vi "gRPC Client Test.vi"() -> ()   [LabVIEW 2021]
uses:
  CIFCore/Common/Typedef/gRPC Reported Plugin Status.ctl
  CIFCore/Common/Typedef/Plugin State.ctl
  CIFCore/Common/Typedef/Timing Statistics.ctl
  CIFCore/Common/Typedef/Timing Stats Base.ctl
  CIFCore/Common/Typedef/FIFO Statistics.ctl
  CIFCore/Common/Typedef/Simple Error.ctl
  CIFCore/Common/Typedef/Monitor Doubles.ctl
  CIFCore/Common/Typedef/Monitor U64.ctl
  CIFCore/Common/Typedef/Monitor I64.ctl
  CIFCore/Common/Typedef/Version.ctl
  CIFCore/Grpc/CIFCorePlugin_client/RPC Messages/cif_plugincore_PluginOverrides.ctl
  CIFCore/Grpc/CIFCorePlugin_client/RPC Messages/cif_plugincore_TimingOverrides.ctl
  CIFCore/Grpc/CIFCorePluginWrapper/CIFCorePluginWrapper.lvlib
  CIFCore/Common/CIFCoreCommon.lvlib
  CIFCore/Grpc/CIFCorePlugin_client/CIFCorePlugin_client.lvlib
panel:
  in  "JSON Configuration 2":string
  in  "stop 2":bool
  out "Plugin Overrides":T1
  out "Version":T3
  out "JSON Configuration":string
  out "Node Status":T4 {"Monitor Doubles"."4" format="%#_9g"; "Monitor Doubles"."3" format="%#_9g"; "Monitor Doubles"."2" format="%#_9g"; "Monitor Doubles"."1" format="%#_9g"}
  in  "change config":bool
  in  "refresh":bool
  in  "stop":bool
  in  "pause":bool
  in  "start":bool
  in  "address":string="192.168.1.160:50051"
  # "Notes to fix.\ngRPC Timing Override\nRemove support for Start FTE"
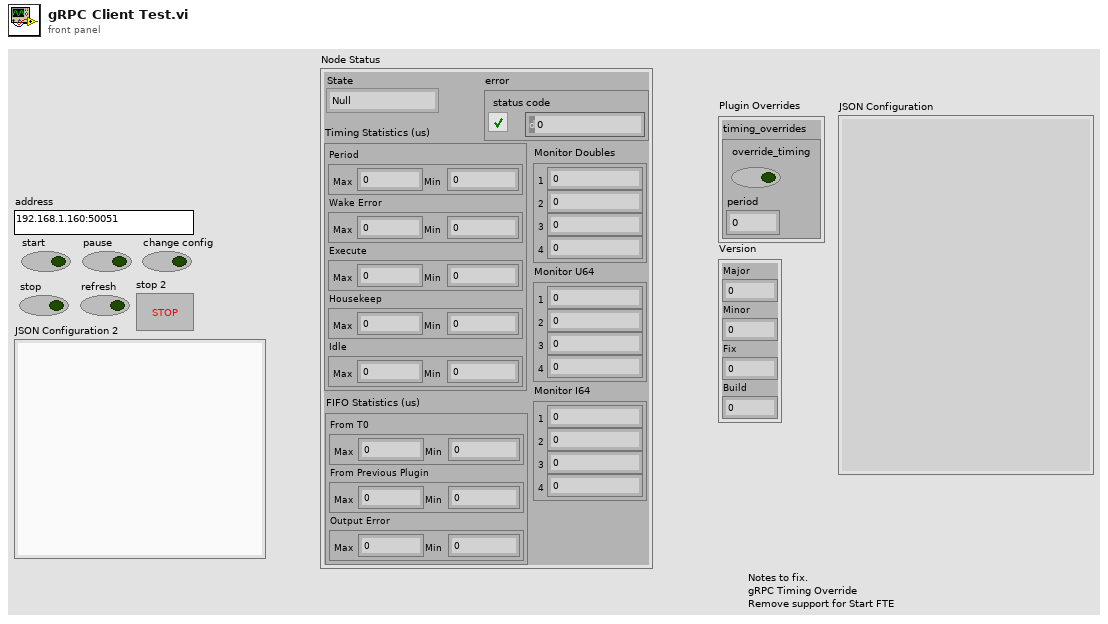
[diagram p1: front panel]
types:
  T1 = typedef "CIFCorePlugin_client.lvlib/cif_plugincore_PluginOverrides.ctl" = cluster{"timing_overrides":T2}
  T2 = typedef "CIFCorePlugin_client.lvlib/cif_plugincore_TimingOverrides.ctl" = cluster{"override_timing":bool, "period":dbl}
  T3 = typedef "CIFCoreCommon.lvlib/Version.ctl" = cluster{"Major":i32, "Minor":i32, "Fix":i32, "Build":i32}
  T4 = typedef "CIFCoreCommon.lvlib/gRPC Reported Plugin Status.ctl" = cluster{"State":T5, "Timing Statistics (us)":T6, "FIFO Statistics (us)":T8, "error":T9, "Monitor Doubles":T10, "Monitor U64":T11, "Monitor I64":T12}
  T5 = typedef "CIFCoreCommon.lvlib/Plugin State.ctl" = enum32{"Null", "Creating", "Listening", "Running", "CleaningUp", "Destroying"}
  T6 = typedef "CIFCoreCommon.lvlib/Timing Statistics.ctl" = cluster{"Period":T7, "Wake Error":T7, "Execute":T7, "Housekeep":T7, "Idle":T7}
  T7 = typedef "CIFCoreCommon.lvlib/Timing Stats Base.ctl" = cluster{"Max":i32, "Min":i32}
  T8 = typedef "CIFCoreCommon.lvlib/FIFO Statistics.ctl" = cluster{"From T0":T7, "From Previous Plugin":T7, "Output Error":T7}
  T9 = typedef "CIFCoreCommon.lvlib/Simple Error.ctl" = cluster{"status":bool, "code":i32}
  T10 = typedef "CIFCoreCommon.lvlib/Monitor Doubles.ctl" = cluster{"1":dbl, "2":dbl, "3":dbl, "4":dbl}
  T11 = typedef "CIFCoreCommon.lvlib/Monitor U64.ctl" = cluster{"1":u64, "2":u64, "3":u64, "4":u64}
  T12 = typedef "CIFCoreCommon.lvlib/Monitor I64.ctl" = cluster{"1":i64, "2":i64, "3":i64, "4":i64}
  T13 = typedef "grpc-lvsupport-release.lvlib/grpcId.ctl" = u64
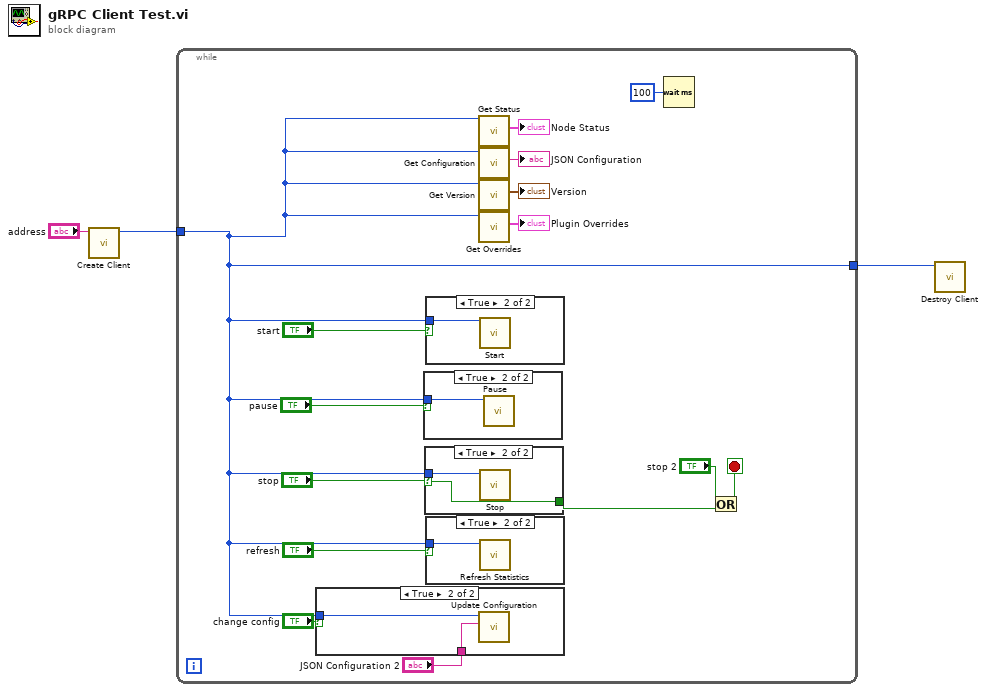
[diagram p0: block diagram]
diagram:
  n1 = call "Create Client.vi"("address"="address") -> ("gRPC ID Out"=w2:T13)  [unwired: 9 in, 1 out]
  n2 = while {
    tunnel: w2 -> [w8]
    tunnel: [w8] -> w1
    stop <- w5 stop-if-true
    n3 = case shown="True" "change config" {
      tunnel: w8 -> [_ w20]
      tunnel: "JSON Configuration 2" -> [_ w19]
      frame False {
      }
      frame True {
        n4 = call "Update Configuration.vi"("JSON Configuration"=w19, "gRPC ID"=w20) -> ()  [unwired: 8 in, 2 out]
      }
    }
    n5 = case shown="True" "pause" {
      tunnel: w8 -> [_ w24]
      frame False {
      }
      frame True {
        n6 = call "Pause.vi"("gRPC ID"=w24) -> ()  [unwired: 9 in, 2 out]
      }
    }
    n7 = case shown="True" "stop" {
      selector: "stop" -> [_ w22]
      tunnel: w8 -> [_ w23]
      tunnel: [_ w22] -> w4
      frame False {
      }
      frame True {
        n8 = call "Stop.vi"("gRPC ID"=w23) -> ()  [unwired: 9 in, 2 out]
      }
    }
    n9 = case shown="True" "start" {
      tunnel: w8 -> [_ w25]
      frame False {
      }
      frame True {
        n10 = call "Start.vi"("gRPC ID"=w25) -> ()  [unwired: 9 in, 2 out]
      }
    }
    n11 = case shown="True" "refresh" {
      tunnel: w8 -> [_ w21]
      frame False {
      }
      frame True {
        n12 = call "Refresh Statistics.vi"("gRPC ID"=w21) -> ()  [unwired: 9 in, 2 out]
      }
    }
    n13 = call "Get Status.vi"("gRPC ID"=w8) -> ("Node Status"=→"Node Status":T4)  [unwired: 8 in, 2 out]
    n14 = call "Get Configuration.vi"("gRPC ID"=w8) -> ("JSON Configuration"=→"JSON Configuration":string)  [unwired: 8 in, 2 out]
    n15 = call "Get Version.vi"("gRPC ID"=w8) -> ("Version"=→"Version":T3)  [unwired: 8 in, 2 out]
    n16 = call "Get Overrides.vi"("gRPC ID"=w8) -> ("Plugin Overrides"=→"Plugin Overrides":T1)  [unwired: 8 in, 2 out]
    n17 = Wait (ms)(milliseconds to wait=u32 100) -> ()  [unwired: 1 out]
    n18 = Or(x="stop 2", y=w4) -> (x .or. y?=w5:bool)
  }
  n19 = call "Destroy Client.vi"("gRPC ID"=w1) -> ()  [unwired: 10 in, 1 out]
